vi "Windows Scan DNS Config.vi"(8 "error in (no error)":errorcluster) -> (0 "error out":errorcluster, 3 "DNS server addresses":refnum<class "Generic Network Address.lvclass">[](array[class]))   [LabVIEW 2020, in "NI_WFCN.lvlib" / "Hostname Network Address.lvclass"]
doc: "Windows: Attempt to locate configured DNS servers."
uses:
  <vilib>/net/WFCN/Addressing/Hostname Network Address/Hostname Network Address.lvclass
  <vilib>/net/WFCN/Addressing/Generic Network Address/Generic Network Address.lvclass
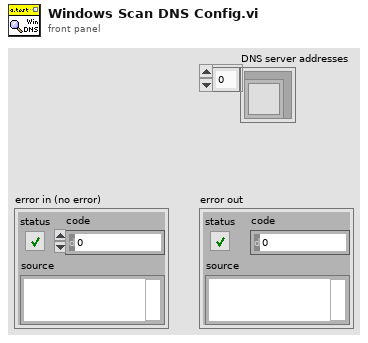
[diagram p1: front panel]
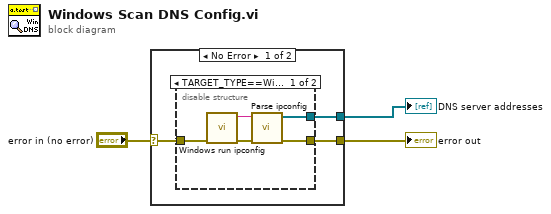
[diagram p0: block diagram]
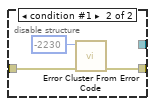
[diagram p2: hidden frame]
diagram:
  n1 = case shown="No Error" "error in (no error)" {
    selector: "error in (no error)" -> [w4 w15]
    tunnel: [w6 w15] -> w3
    tunnel: [w5 _] -> w2
    frame No Error {
      n2 = disable-structure shown="TARGET_TYPE==Windows" {
        disable-tunnel: [w11 w12] -> w6
        disable-tunnel: [w9 _] -> w5
        disable-tunnel: w4 -> [w7 w13]
        frame condition #0 (active) {
          n3 = call <vilib>:"Windows run ipconfig.vi"("error in (no error)"=w7) -> ("error out"=w10:errorcluster, "standard output"=w8:string)  [unwired: 9 in]
          n4 = call <vilib>:"Parse ipconfig.vi"("error in (no error)"=w10, "ipconfig stdout"=w8) -> ("error out"=w11:errorcluster, "DNS server addresses"=w9:refnum<class "Generic Network Address.lvclass">[])  [unwired: 8 in]
        }
        frame condition #1 {
          n5 = call <vilib>:"Error Cluster From Error Code.vi"("error in (no error)"=w13, "error code (0)"=-2230 ("\"This VI is not supported on the current platform\"")) -> ("error out"=w12:errorcluster)  [unwired: 7 in]
        }
      }
    }
    frame Error {
    }
  }
  "error out" <- w3
  "DNS server addresses" <- w2
